vi "Pre Launch Init.vi"(11 "Async Actor Example in":refnum<class "Async Methods Actor Example.lvclass">) -> (0 "error out":errorcluster, 3 "Async Actor Example out":refnum<class "Async Methods Actor Example.lvclass">)   [LabVIEW 2021, in "Async Methods Actor Example.lvlib" / "Async Methods Actor Example.lvclass"]
doc: "(<B>Filename</B>: Actor Framework.lvlib:Actor.lvclass:Pre Launch Init.vi)\n\nDefines behavior that occurs after the Launch Nested Actor method is invoked but before the actor's Actor Core method begins running.\n\nBy default, this method does nothing. A descendant class may override it to define behavior."
uses:
  Async Methods Actor Example.lvclass
  Async Methods Actor/Async Methods Actor Messages/Completion Notification Msg/Completion Notification Data.ctl
  Async Methods Actor/Async Methods Actor Messages/Async Message/Async Message.lvclass
  Async Methods Actor Example.lvclass/Async Methods Actor Example.ctl
  Async Methods Actor/Async Methods Actor/Async Methods Actor.lvclass
  Async Methods Actor/Async Methods Actor Messages/Completion Notification Msg/Completion Notification Msg.lvclass
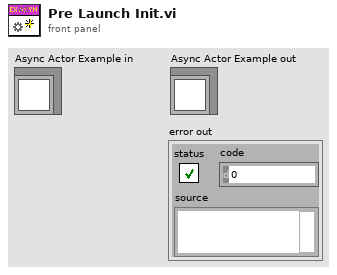
[diagram p1: front panel]
types:
  T1 = typedef "Async Methods Actor.lvlib/Completion Notification Msg.lvclass/Completion Notification Data.ctl" = cluster{"Async Message":refnum<class "Async Message.lvclass">, "Current Execution Count":u32}
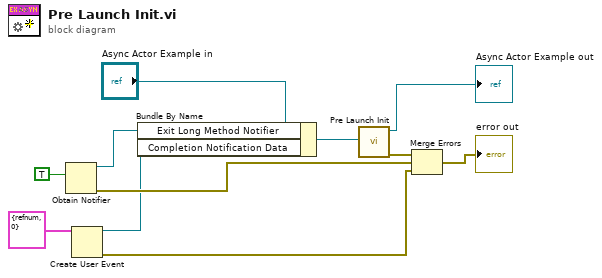
[diagram p0: block diagram]
diagram:
  n1 = Obtain Notifier(notification data type=TRUE) -> (notifier out=w6:refnum<notifier>, error out=w4:errorcluster)  [unwired: 3 in, 1 out]
  n2 = Create User Event(user event datatype=T1 {"Async Message"=refnum, "Current Execution Count"=0} ("Completion Ack Data")) -> (user event=w1:refnum<user-event>, error out=w2:errorcluster)  [unwired: 1 in]
  n3 = Bundle By Name(cluster="Async Actor Example in", "Exit Long Method Notifier"=w6, "Completion Notification Data"=w1) -> (w7:refnum<class "Async Methods Actor Example.lvclass">)
  n4 = call-parent "Pre Launch Init.vi"("Async Methods Actor in"=w7) -> ("error out"=w11:errorcluster, "Async Methods Actor out"=→"Async Actor Example out":refnum<class "Async Methods Actor Example.lvclass">)  [unwired: 9 in]
  n5 = Merge Errors(w11, w4, w2) -> (→"error out":errorcluster)
